vi "limitVSent.vi"(10 "MaxVSent":dbl, 11 "Robot in":refnum<class "Robot.lvclass">) -> (3 "Robot out":refnum<class "Robot.lvclass">)   [LabVIEW 2021, in "Robot.lvclass"]
uses:
  Robot.lvclass
  tactics.ctl
  Robot.lvclass/Robot.ctl
  <vilib>/Analysis/_algsub.llb/Real Vector Norm.vi
  <vilib>/Analysis/baseanly.llb/Unit Vector (DBL).vi
  Write v_tang.vi
  Write v_norm.vi
  Read v_tang.vi
  Read v_norm.vi
  Read tactic.vi
  <vilib>/Analysis/NI_AALPro.lvlib
  <vilib>/Analysis/NI_AALBase.lvlib
panel:
  out "error out":errorcluster
  in  "error in (no error)":errorcluster
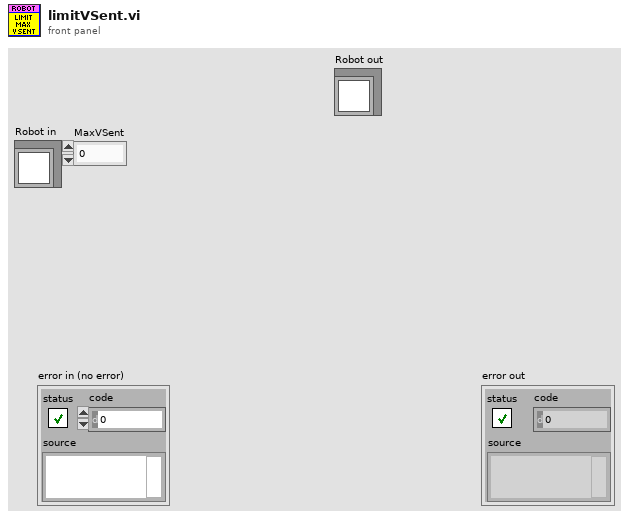
[diagram p1: front panel]
types:
  T1 = typedef "tactics.ctl" = enum16{"GoToBallPlacementPosition", "PlaceBall", "GoToBallPlacement", "5Robots", "BallPlacementEnemy", "ReceivePassInFuturePoint", "Roller", "PrepareRollToPassRollerGoTo", "PrepareRollToPassReceiverGoTo", "WaitRoll", "PositionToRoll", "PenaltyAttacker", "PassObserver", "PenaltyDefense", "TableReceiverTactic", "Test", "DefendGoal", "Marker", "FollowAttacker", "DefendArea", "Shoot", "AttackerAimGoal", "AttackerBallOutOfField", "AttackerBlock", "AttackerStop", "Duelist", "Halt", "ZigZag", "GoTo", "Timeout", "KickToBestRobot", "KickToPassReceiver", "PositionToReceivePass", "WaitPass"}
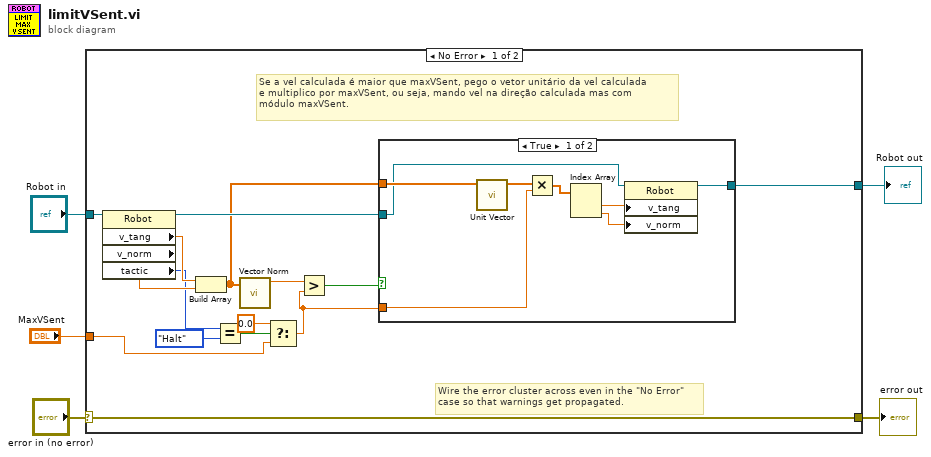
[diagram p0: block diagram]
diagram:
  n1 = case shown="No Error" "error in (no error)" {
    selector: "error in (no error)" -> [w20 w30]
    tunnel: [w20 w30] -> w4
    tunnel: "Robot in" -> [w17 _]
    tunnel: "MaxVSent" -> [w6 _]
    tunnel: [w13 _] -> w1
    frame No Error {
      # "Se a vel calculada é maior que maxVSent, pego o vetor unitário da vel calculada\ne multiplico por maxVSent, ou seja, mando vel na direção calculada mas com\nmódulo maxVSent."
      # "Wire the error cluster across even in the \"No Error\"\ncase so that warnings get propagated."
      n2 = property class="Robot"(reference=w17) -> (reference out=w14:refnum<class "Robot.lvclass">, "v_tang"=w16:dbl, "v_norm"=w15:dbl, "tactic"=w11:T1)  [unwired: 1 in, 1 out]
      n3 = Build Array(w16, w15) -> (w12:dbl[])
      n4 = Equal?(x=w11, y=tactics."Halt") -> (x = y?=w9:bool)
      n5 = call-poly <vilib>:"Vector Norm.vi"("Input Vector"=w12) -> ("norm"=w18:dbl)  [unwired: 9 in, 1 out]
      n6 = Select(t=0.0, s=w9, f=w6) -> (s? t:f=w7:dbl)
      n7 = Greater?(x=w18, y=w7) -> (0:w19:bool)
      n8 = case shown="True" w19 {
        tunnel: [w28 w29] -> w13
        tunnel: w14 -> [w21 w29]
        tunnel: w12 -> [w23 _]
        tunnel: w7 -> [w22 _]
        frame True {
          n9 = call-poly <vilib>:"Unit Vector.vi"("Input Vector"=w23) -> ("Unit Vector"=w27:dbl[])  [unwired: 8 in, 2 out]
          n10 = Multiply(x=w27, y=w22) -> (x*y=w26:dbl[])
          n11 = Index Array(array=w26) -> (element #1=w25:dbl, element #2=w24:dbl)  [unwired: 2 in]
          n12 = property class="Robot"(reference=w21, "v_tang"=w25, "v_norm"=w24) -> (reference out=w28:refnum<class "Robot.lvclass">)  [unwired: 1 in, 1 out]
        }
        frame False {
        }
      }
    }
    frame Error {
    }
  }
  "error out" <- w4
  "Robot out" <- w1
